vi "mainV2.vi"() -> ()   [LabVIEW 2020]
uses:
  node_type.ctl
  node.ctl
  d2cbbd9a-39bd-4934-8608-8b79aaeda0e4.vi
  <vilib>/JDP Science/JSONtext/Variant to JSON Text.vi
  <vilib>/JDP Science/JSONtext/LVClass Serializer/JSONtext LVClass Serializer.lvclass
panel:
  in  "文件路径（使用对话框）":path=path "C:/Users/Fred/Desktop/LabAI/data/main.json"
  out "json_output":string
  out "分析时间":dbl format="%.3f s"
  in  "Path to Entrance VI":path=path "C:/Users/Fred/Desktop/LabAI/mainV2.vi"
  # "C:\\Users\\Fred\\Desktop\\LabAI\\mainV2.vi"
  # "C:\\Users\\Fred\\Desktop\\FL62风洞主控软件\\Desktop\\2.4米风洞主控软件20240716\\主程序 - 一键启动-web.vi"
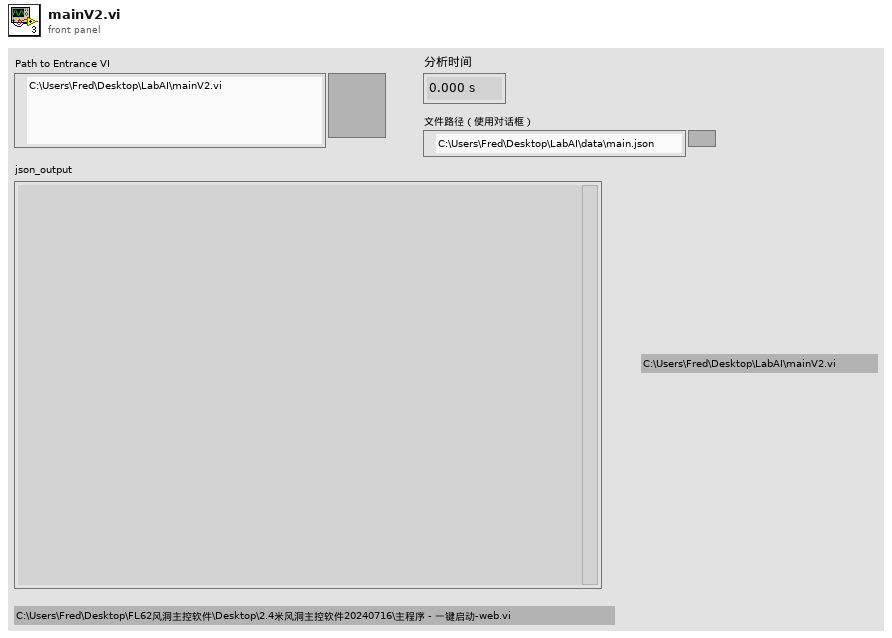
[diagram p1: front panel]
types:
  T1 = typedef "node.ctl" = cluster{"id":string, "VIName":string, "VIPath":string, "type":string, "label":string, "parentId":string, "nodes":variant[], "frames":variant[], "properties":variant[], "metadata":variant[]}
  T2 = typedef "node_type.ctl" = enum16{"VI", "SubVI", "Function", "ForLoop", "WhileLoop", "Frame", "CaseStructure", "EventStructure"}
  T3 = enum16{"open", "replace", "create", "open or create", "replace or create", "replace or create with confirmation"}
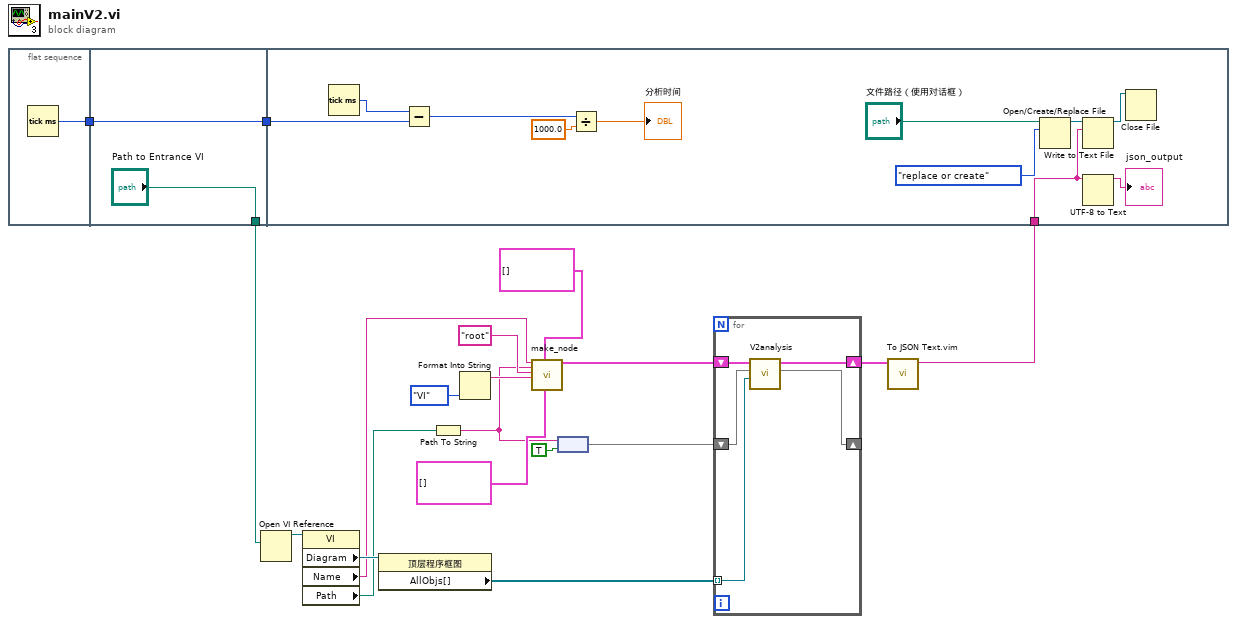
[diagram p0: block diagram]
diagram:
  n1 = flat-sequence {
    tunnel: [w20] -> w19
    tunnel: ["Path to Entrance VI"] -> w13
    tunnel: w19 -> [w21]
    tunnel: [w21] -> w18
    tunnel: w18 -> [w32]
    tunnel: w2 -> [w24]
    frame #0 {
      n2 = Tick Count (ms)() -> (millisecond timer value=w20:u32)
    }
    frame #1 {
    }
    frame #2 {
      n3 = Tick Count (ms)() -> (millisecond timer value=w33:u32)
      n4 = Subtract(x=w33, y=w32) -> (x-y=w30:u32)
      n5 = Divide(x=w30, y=1000.0) -> (x/y=→"分析时间":dbl)
      n6 = Open/Create/Replace File(file path (use dialog)="文件路径（使用对话框）", operation (0:open)=T3."replace or create" ("操作(0:open)")) -> (refnum out=w26:refnum<file>)  [unwired: 4 in, 2 out]
      n7 = Write to Text File(file (use dialog)=w26, text=w24) -> (refnum out=w25:refnum<file>)  [unwired: 2 in, 2 out]
      n8 = UTF-8 to Text(11:w24) -> (3:→"json_output":string)  [unwired: 2 in, 1 out]
      n9 = Close File(refnum=w25) -> ()  [unwired: 1 in, 2 out]
    }
  }
  n10 = Open VI Reference(vi path=w13) -> (vi reference=w17:refnum<vi>)  [unwired: 5 in, 1 out]
  n11 = property class="VI"(reference=w17) -> ("Diagram"=w16:refnum<vi>, "Name"=w12:string, "Path"=w14:path)  [unwired: 1 in, 2 out]
  n12 = property class="顶层程序框图"(reference=w16) -> ("AllObjs[]"=w15:refnum<vi>[])  [unwired: 1 in, 2 out]
  n13 = Path To String(path=w14) -> (string=w6:string)
  n14 = Format Into String(node_type."VI" ("枚举")) -> (resulting string=w9:string)  [unwired: 3 in, 1 out]
  n15 = call "make_node.vi"("VIName"=w12, "VIPath"=w6, "id"="root", "type"=w9, "frames"=T1[] [] ("nodes"), "nodes"=T1[] []) -> ("node"=w7:T1)  [unwired: 13 in]
  n16 = node(w6, TRUE) -> (w4:map{string, bool})
  n17 = for {
    tunnel: w15 -> [w38] mode=indexing
    shift-right: [w35] -> _
    shift-left: w4 -> [w36]
    shift-right: [w34] -> w3
    shift-left: w7 -> [w37]
    n18 = call "V2analysis.vi"("node_in"=w37, "VIPathMap"=w36, "GObj引用句柄"=w38) -> ("node_out"=w34:T1, "VIPathMap 2"=w35:map{string, bool})  [unwired: 6 in]
  }
  n19 = call "To JSON Text.vim"("Anything"=w3) -> ("<JSON>"=w2:string)  [unwired: 9 in, 1 out]
